vi "Autonomous Independent.vi"() -> ()   [LabVIEW 2014]
doc: "This VI is called when autonomous begins, and will automatically be terminated when autonomous ends. You can carry out timed or sensor driven robot movement independently without needing to return to the caller."
uses:
  Robot Global Data.vi
  <vilib>/Rock Robotics/WPI/RobotDrive/WPI_RobotDriveMecanumDrive_Cartesian.vi
  <vilib>/Rock Robotics/Network Tables/SD Write Numeric Array.vi
panel:
  in  "Instructions":T1(array[cluster])
  out "Current Movement, for debugging":T2 {"Z Joystick Value" scale=-1.0..1.0; "Y Joystick Value" scale=1.0..-1.0; "X Joystick Value" scale=-1.0..1.0}
  in  "Array of robot movements":T3(array[cluster]) {"Z Joystick Value" scale=-1.0..1.0; "Y Joystick Value" scale=1.0..-1.0; "X Joystick Value" scale=-1.0..1.0}
  # "Be sure to right-click and choose Data Operations>>Make Current Value default if you want to save the array values with the VI"
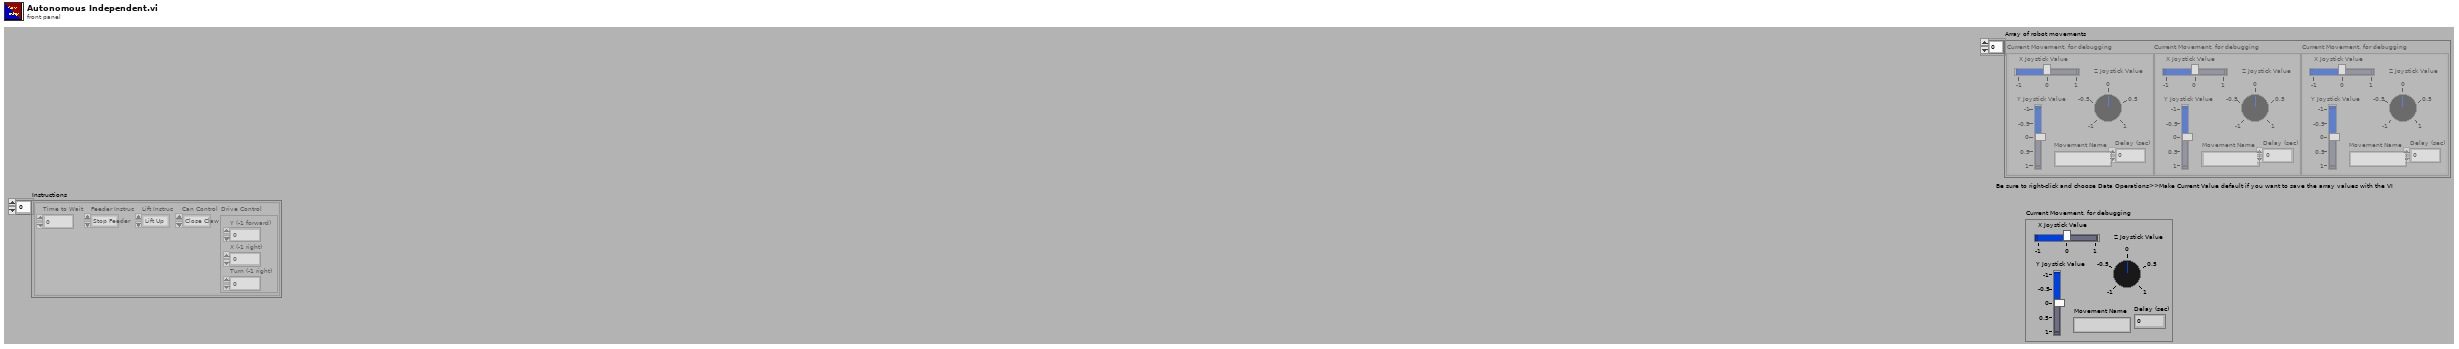
[diagram p1: front panel]
types:
  T1 = cluster{"Time to Wait":dbl, "Feeder Instruc":enum16{"Stop Feeder", "Infeed", "Outfeed", "Rightfeed", "Leftfeed"}, "Lift Instruc":enum16{"Lift Up", "Lift Down"}, "Can Control":enum16{"Close Claw", "Open Claw", "Fast Up", "Slow Up", "Stop", "Srow Down", "Fast Down"}, "Drive Control":cluster{"Y (-1 forward) ":dbl, "X (-1 right)":dbl, "Turn (-1 right)":dbl}}[]
  T2 = cluster{"X Joystick Value":dbl, "Y Joystick Value":dbl, "Z Joystick Value":dbl, "Delay (sec)":dbl, "Movement Name":string}
  T3 = cluster{"X Joystick Value":dbl, "Y Joystick Value":dbl, "Z Joystick Value":dbl, "Delay (sec)":dbl, "Movement Name":string}[]
  T4 = enum16{"open", "replace", "create", "open or create", "replace or create", "replace or create with confirmation"}
  T5 = cluster{"Time to Start":dbl, "Action":enum16{"Stop", "Drive Forward", "Drive Backwards", "Turn Right", "Turn Left", "Tote Up", "Tote Down", "Doors Open", "Doors Close", "Claw Open", "Claw Close", "Claw Up", "Claw Down", "Infeed In", "Infeed Out", "Infeed Off"}}[]
  T6 = typedef "WPI_RobotDriveDevRef.ctl" = cluster{"DevStatus":errorcluster, "Motors[]":T7[], "Square Inputs":bool, "Max Output":dbl}
  T7 = typedef "WPI_MotorControlDeviceRef.ctl" = cluster{"DeviceStatus":errorcluster, "Type":T8, "PWM":cluster{"Controller":T9, "PWM Channel":T10, "DeadBand":T11}, "CAN":cluster{"Device Number":u8, "Control Mode":T12, "Semaphore":T13, "Max Vout":dbl, "TalonSRX Control Mode":T14}, "Invert":bool, "TransformRef":T15, "InvTransformRef":T15}
  T8 = typedef "WPI_MotorControlType.ctl" = enum16{"PWM", "CAN", "CANTalonSRX"}
  T9 = typedef "FPGA_TypedefDigitalModule.ctl" = enum16{"Controller 1"}
  T10 = typedef "FPGA_DIOPWMChannel.ctl" = enum8{"PWM 0", "PWM 1", "PWM 2", "PWM 3", "PWM 4", "PWM 5", "PWM 6", "PWM 7", "PWM 8", "PWM 9", "PWM MXP 0", "PWM MXP 1", "PWM MXP 2", "PWM MXP 3", "PWM MXP 4", "PWM MXP 5", "PWM MXP 6", "PWM MXP 7", "PWM MXP 8", "PWM MXP 9", "Invalid"}
  T11 = typedef "WPI_PWMDeadband.ctl" = cluster{"Name":string, "maxPositivePwm":i32, "minPositivePwm":i32, "centerPwm":i32, "maxNegativePwm":i32, "minNegativePwm":i32, "angularRange":u16}
  T12 = typedef "WPI_CANJaguar_ControlMode.ctl" = enum8{"Percent VBus", "Current", "Speed", "Position", "Voltage"}
  T13 = typedef "Semaphore RefNum" = refnum<k1>
  T14 = typedef "WPI_CANTalonSRX_APIControlMode.ctl" = enum8{"Percent VBus", "Speed", "Position", "Slave", "Unchanged / Invalid"}
  T15 = typedef "WPI_PWMTransform_ConPane.ctl" = refnum<vi>
  T16 = enum16{"Stop Feeder", "Infeed", "Outfeed", "Rightfeed", "Leftfeed"}
  T17 = enum16{"Close Claw", "Open Claw", "Fast Up", "Slow Up", "Stop", "Srow Down", "Fast Down"}
  T18 = cluster{"Y (-1 forward) ":dbl, "X (-1 right)":dbl, "Turn (-1 right)":dbl}
  T19 = cluster{"Lifter Down":bool, "Right Infeed":enum16{"Off", "Forward", "Reverse"}, "Left Infeed":enum16{"Off", "Forward", "Reverse"}}
  T20 = cluster{"Motor Speed":dbl, "Grabber":bool, "Go Up a Level":bool, "Go Down a Level":bool}
  T21 = typedef "Rendezvous RefNum" = refnum<k1>
  T22 = enum16{"Stop", "Drive Forward", "Drive Backwards", "Turn Right", "Turn Left", "Tote Up", "Tote Down", "Doors Open", "Doors Close", "Claw Open", "Claw Close", "Claw Up", "Claw Down", "Infeed In", "Infeed Out", "Infeed Off"}
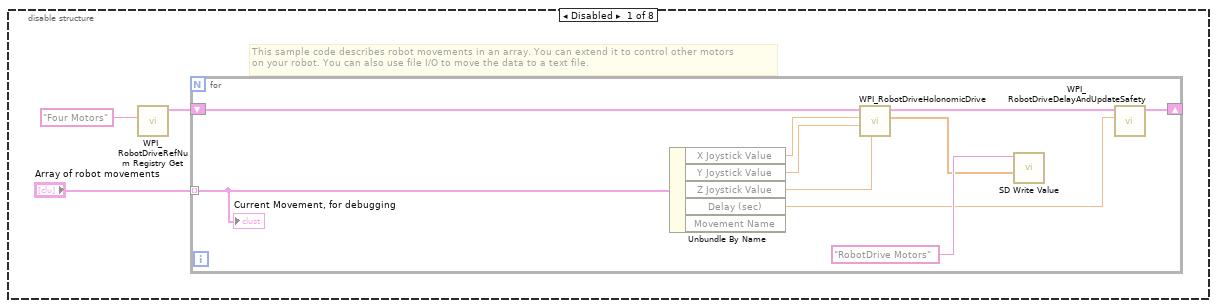
[diagram p2: hidden frame]
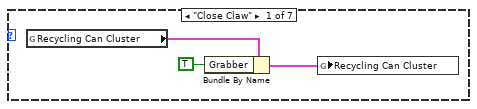
[diagram p3: hidden frame]
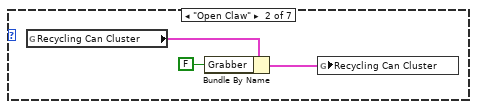
[diagram p4: hidden frame]
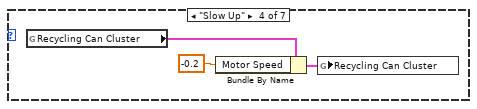
[diagram p5: hidden frame]
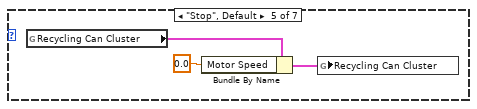
[diagram p6: hidden frame]
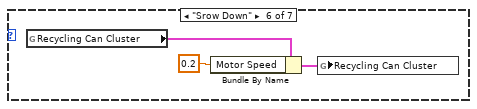
[diagram p7: hidden frame]
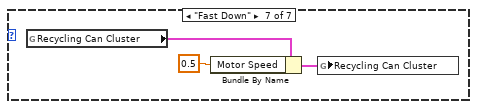
[diagram p8: hidden frame]
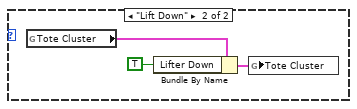
[diagram p9: hidden frame]
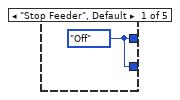
[diagram p10: hidden frame]
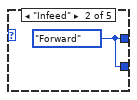
[diagram p11: hidden frame]
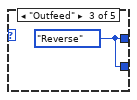
[diagram p12: hidden frame]
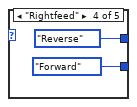
[diagram p13: hidden frame]
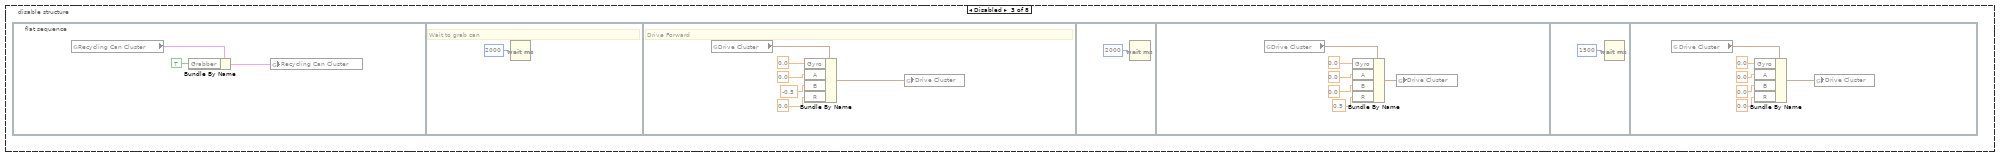
[diagram p14: hidden frame]
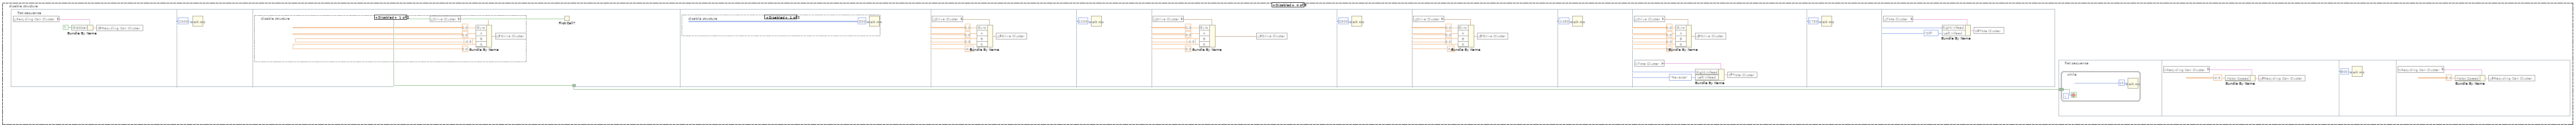
[diagram p15: hidden frame]
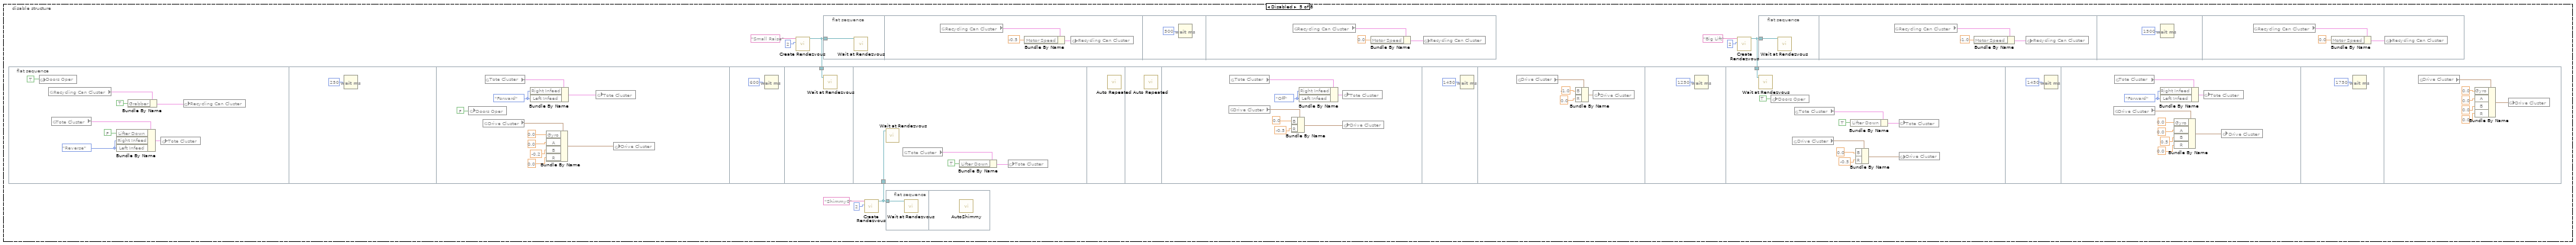
[diagram p18: hidden frame]
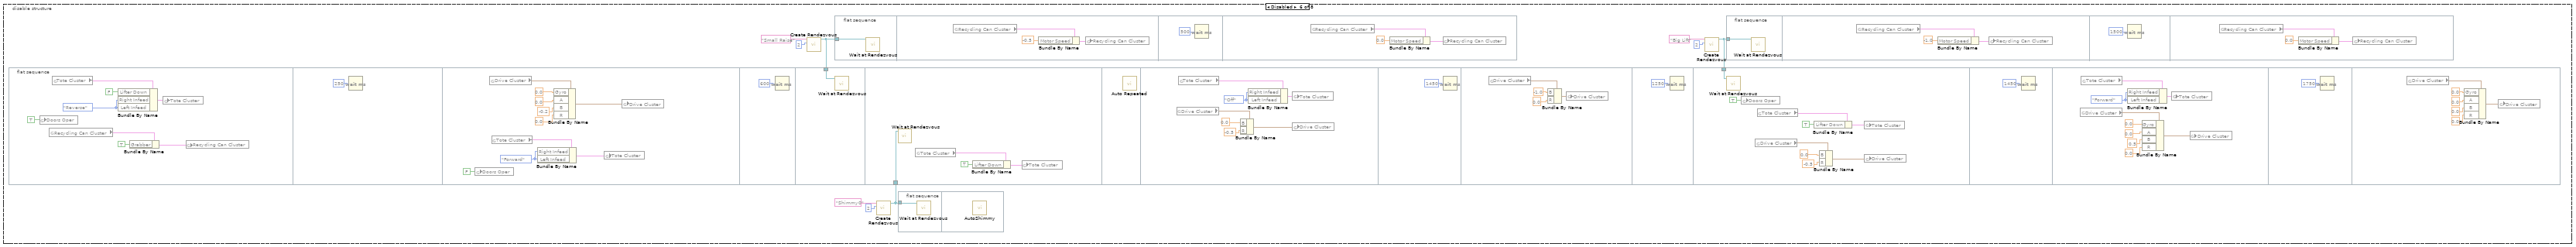
[diagram p19: hidden frame]
diagram:
  # "Every 20ms, report that we are running autonomous\ncode. Loop will abort the same time as the VI."
  # "This tells you the driver position\nand alliance color"
  n1 = call <vilib>:"WPI_DriverStationGet Alliance Info.vi"() -> ()  [unwired: 12 out]
  n2 = disable-structure shown="Enabled" {
    frame Disabled {
      # "This sample code describes robot movements in an array. You can extend it to control other motors\non your robot. You can also use file I/O to move the data to a text file."
      n3 = call <vilib>:"WPI_RobotDriveRefNum Registry Get.vi"("refnum name"="Four Motors") -> ("RobotDriveDevRef"=w2:T6)  [unwired: 1 in, 9 out]
      n4 = for {
        shift-right: [w10] -> _
        shift-left: w2 -> [w11]
        tunnel: "Array of robot movements" -> [w6] mode=indexing
        n5 = Unbundle By Name(w6) -> ("X Joystick Value"=w9:dbl, "Y Joystick Value"=w8:dbl, "Z Joystick Value"=w5:dbl, "Delay (sec)"=w7:dbl)  [unwired: 1 out]
        n6 = call-poly <vilib>:"WPI_RobotDriveHolonomicDrive.vi"("Rotation"=w5, "Y"=w8, "X"=w9, "RobotDriveDevRef"=w11) -> ("Motor Values"=w4:dbl[], "RobotDriveDevRef"=w12:T6)  [unwired: 5 in, 1 out]
        n7 = call-poly <vilib>:"SD Write Value.vi"("Numeric Array"=w4, "Name"="RobotDrive Motors") -> ()  [unwired: 8 in, 2 out]
        n8 = call <vilib>:"WPI_RobotDriveDelayAndUpdateSafety.vi"("Delay (s)"=w7, "RobotDriveDevRef"=w12) -> ("RobotDriveDevRef 2"=w10:T6)  [unwired: 8 in, 1 out]
        "Current Movement, for debugging" <- w6
      }
    }
    frame Enabled {
      n9 = Current VI's Path() -> (path=w21:path)
      n10 = Strip Path(path=w21) -> (stripped path=w22:path)  [unwired: 1 out]
      n11 = Build Path(base path=w22, name or relative path="auto.instruct") -> (appended path=w19:path)
      n12 = Open/Create/Replace File(file path (use dialog)=w19, operation (0:open)=T4."open", access (0:read/write)=enum16{"read/write", "read-only", "write-only"}."read-only") -> (refnum out=w18:refnum<file>)  [unwired: 3 in, 2 out]
      n13 = Read from Text File(file (use dialog)=w18) -> (text=w17:string)  [unwired: 3 in, 3 out]
      n14 = Unflatten From String(type="Instructions", binary string=w17) -> (value=w16:T1)  [unwired: 3 in, 2 out]
      n15 = Array Size(array=w16) -> (size(s)=w20:i32)
      n16 = Tick Count (ms)() -> (millisecond timer value=w14:u32)
      n17 = for {
        N: w20 -> [_]
        tunnel: w16 -> [w32] mode=indexing
        tunnel: w14 -> [w26]
        n18 = Unbundle By Name(w32) -> ("Time to Wait"=w31:dbl, "Feeder Instruc"=w29:T16, "Lift Instruc"=w28:enum16{"Lift Up", "Lift Down"}, "Can Control"=w27:T17, "Drive Control"=w30:T18)
        n19 = flat-sequence {
          tunnel: w31 -> [w33]
          tunnel: w26 -> [w34]
          tunnel: w30 -> [w44]
          tunnel: w29 -> [w43]
          tunnel: w28 -> [w42]
          tunnel: w27 -> [w41]
          frame #0 {
            n20 = while {
              tunnel: w34 -> [w39]
              tunnel: w33 -> [w37]
              stop <- w36 stop-if-true
              n21 = Tick Count (ms)() -> (millisecond timer value=w40:u32)
              n22 = Subtract(x=w40, y=w39) -> (x-y=w38:u32)
              n23 = Greater?(x=w38, y=w37) -> (0:w36:bool)
              n24 = Wait (ms)(milliseconds to wait=u32 5) -> ()  [unwired: 1 out]
            }
          }
          frame #1 {
            n25 = flat-sequence "Feeder Control" {
              tunnel: w43 -> [w78]
              frame #0 {
                n26 = case shown="\"Leftfeed\"" w78 {
                  tunnel: [w79 w80 w81 enum16{"Off", "Forward", "Reverse"}."Reverse" ("Right Infeed") enum16{"Off", "Forward", "Reverse"}."Forward" ("Right Infeed")] -> w75
                  tunnel: [w79 w80 w81 enum16{"Off", "Forward", "Reverse"}."Forward" ("Right Infeed") enum16{"Off", "Forward", "Reverse"}."Reverse" ("Right Infeed")] -> w74
                  frame "Stop Feeder", Default {
                    w79 = enum16{"Off", "Forward", "Reverse"}."Off" ("Right Infeed")
                  }
                  frame "Infeed" {
                    w80 = enum16{"Off", "Forward", "Reverse"}."Forward" ("Right Infeed")
                  }
                  frame "Outfeed" {
                    w81 = enum16{"Off", "Forward", "Reverse"}."Reverse" ("Right Infeed")
                  }
                  frame "Rightfeed" {
                  }
                  frame "Leftfeed" {
                  }
                }
                n27 = global read "Robot Global Data.vi" "Tote Cluster"() -> (w77:T19)
                n28 = Bundle By Name(cluster=w77, "Right Infeed"=w75, "Left Infeed"=w74) -> (w76:T19)
                n29 = global write "Robot Global Data.vi" "Tote Cluster"(w76) -> ()
              }
            }
            n30 = flat-sequence "Lift Instruc" {
              tunnel: w42 -> [w67]
              frame #0 {
                n31 = case shown="\"Lift Up\", Default" w67 {
                  frame "Lift Up", Default {
                    n32 = global read "Robot Global Data.vi" "Tote Cluster"() -> (w70:T19)
                    n33 = Bundle By Name(cluster=w70, "Lifter Down"=FALSE) -> (w69:T19)
                    n34 = global write "Robot Global Data.vi" "Tote Cluster"(w69) -> ()
                  }
                  frame "Lift Down" {
                    n35 = global read "Robot Global Data.vi" "Tote Cluster"() -> (w73:T19)
                    n36 = Bundle By Name(cluster=w73, "Lifter Down"=TRUE) -> (w72:T19)
                    n37 = global write "Robot Global Data.vi" "Tote Cluster"(w72) -> ()
                  }
                }
              }
            }
            n38 = flat-sequence "Claw Instruc" {
              tunnel: w41 -> [w45]
              frame #0 {
                n39 = case shown="\"Fast Up\"" w45 {
                  frame "Close Claw" {
                    n40 = global read "Robot Global Data.vi" "Recycling Can Cluster"() -> (w48:T20)
                    n41 = Bundle By Name(cluster=w48, "Grabber"=TRUE) -> (w47:T20)
                    n42 = global write "Robot Global Data.vi" "Recycling Can Cluster"(w47) -> ()
                  }
                  frame "Open Claw" {
                    n43 = global read "Robot Global Data.vi" "Recycling Can Cluster"() -> (w51:T20)
                    n44 = Bundle By Name(cluster=w51, "Grabber"=FALSE) -> (w50:T20)
                    n45 = global write "Robot Global Data.vi" "Recycling Can Cluster"(w50) -> ()
                  }
                  frame "Fast Up" {
                    n46 = global read "Robot Global Data.vi" "Recycling Can Cluster"() -> (w54:T20)
                    n47 = Bundle By Name(cluster=w54, "Motor Speed"=-0.5) -> (w53:T20)
                    n48 = global write "Robot Global Data.vi" "Recycling Can Cluster"(w53) -> ()
                  }
                  frame "Slow Up" {
                    n49 = global read "Robot Global Data.vi" "Recycling Can Cluster"() -> (w57:T20)
                    n50 = Bundle By Name(cluster=w57, "Motor Speed"=-0.2) -> (w56:T20)
                    n51 = global write "Robot Global Data.vi" "Recycling Can Cluster"(w56) -> ()
                  }
                  frame "Stop", Default {
                    n52 = global read "Robot Global Data.vi" "Recycling Can Cluster"() -> (w60:T20)
                    n53 = Bundle By Name(cluster=w60, "Motor Speed"=0.0) -> (w59:T20)
                    n54 = global write "Robot Global Data.vi" "Recycling Can Cluster"(w59) -> ()
                  }
                  frame "Srow Down" {
                    n55 = global read "Robot Global Data.vi" "Recycling Can Cluster"() -> (w63:T20)
                    n56 = Bundle By Name(cluster=w63, "Motor Speed"=0.2) -> (w62:T20)
                    n57 = global write "Robot Global Data.vi" "Recycling Can Cluster"(w62) -> ()
                  }
                  frame "Fast Down" {
                    n58 = global read "Robot Global Data.vi" "Recycling Can Cluster"() -> (w66:T20)
                    n59 = Bundle By Name(cluster=w66, "Motor Speed"=0.5) -> (w65:T20)
                    n60 = global write "Robot Global Data.vi" "Recycling Can Cluster"(w65) -> ()
                  }
                }
              }
            }
            n61 = flat-sequence "Drive Instruction" {
              tunnel: w44 -> [w91]
              frame #0 {
                n62 = Unbundle By Name(w91) -> ("Y (-1 forward)"=w90:dbl, "X (-1 right)"=w89:dbl, "Turn (-1 right)"=w88:dbl)
                n63 = global read "Robot Global Data.vi" "Drive Cluster"() -> (w87:cluster{"A":dbl, "B":dbl, "R":dbl, "Gyro":dbl})
                n64 = Bundle By Name(cluster=w87, "A"=w89, "B"=w90, "R"=w88) -> (w86:cluster{"A":dbl, "B":dbl, "R":dbl, "Gyro":dbl})
                n65 = global write "Robot Global Data.vi" "Drive Cluster"(w86) -> ()
              }
            }
          }
        }
      }
    }
    frame Disabled {
      n66 = flat-sequence {
        frame #0 {
          n67 = global read "Robot Global Data.vi" "Recycling Can Cluster"() -> (w93:T20)
          n68 = Bundle By Name(cluster=w93, "Grabber"=TRUE) -> (w92:T20)
          n69 = global write "Robot Global Data.vi" "Recycling Can Cluster"(w92) -> ()
        }
        frame #1 {
          # "Wait to grab can"
          n70 = Wait (ms)(milliseconds to wait=u32 2000) -> ()  [unwired: 1 out]
        }
        frame #2 {
          # "Drive Forward"
          n71 = global read "Robot Global Data.vi" "Drive Cluster"() -> (w101:cluster{"A":dbl, "B":dbl, "R":dbl, "Gyro":dbl})
          n72 = Bundle By Name(cluster=w101, "Gyro"=0.0, "A"=0.0, "B"=-0.5, "R"=0.0) -> (w100:cluster{"A":dbl, "B":dbl, "R":dbl, "Gyro":dbl})
          n73 = global write "Robot Global Data.vi" "Drive Cluster"(w100) -> ()
        }
        frame #3 {
          n74 = Wait (ms)(milliseconds to wait=u32 2000 ("millisecond multiple")) -> ()  [unwired: 1 out]
        }
        frame #4 {
          n75 = global read "Robot Global Data.vi" "Drive Cluster"() -> (w103:cluster{"A":dbl, "B":dbl, "R":dbl, "Gyro":dbl})
          n76 = Bundle By Name(cluster=w103, "Gyro"=0.0, "A"=0.0, "B"=0.0, "R"=0.5) -> (w104:cluster{"A":dbl, "B":dbl, "R":dbl, "Gyro":dbl})
          n77 = global write "Robot Global Data.vi" "Drive Cluster"(w104) -> ()
        }
        frame #5 {
          n78 = Wait (ms)(milliseconds to wait=u32 1500 ("millisecond multiple")) -> ()  [unwired: 1 out]
        }
        frame #6 {
          n79 = global read "Robot Global Data.vi" "Drive Cluster"() -> (w110:cluster{"A":dbl, "B":dbl, "R":dbl, "Gyro":dbl})
          n80 = Bundle By Name(cluster=w110, "Gyro"=0.0, "A"=0.0, "B"=0.0, "R"=0.0) -> (w111:cluster{"A":dbl, "B":dbl, "R":dbl, "Gyro":dbl})
          n81 = global write "Robot Global Data.vi" "Drive Cluster"(w111) -> ()
        }
      }
    }
    frame Disabled {
      n82 = flat-sequence {
        tunnel: [w131] -> w116
        frame #0 {
          n83 = global read "Robot Global Data.vi" "Recycling Can Cluster"() -> (w128:T20)
          n84 = Bundle By Name(cluster=w128, "Grabber"=TRUE) -> (w127:T20)
          n85 = global write "Robot Global Data.vi" "Recycling Can Cluster"(w127) -> ()
        }
        frame #1 {
          n86 = Wait (ms)(milliseconds to wait=u32 2000) -> ()  [unwired: 1 out]
        }
        frame #2 {
          n87 = disable-structure shown="Disabled" {
            frame Disabled {
              n88 = global read "Robot Global Data.vi" "Drive Cluster"() -> (w137:cluster{"A":dbl, "B":dbl, "R":dbl, "Gyro":dbl})
              n89 = Bundle By Name(cluster=w137, "Gyro"=0.0, "A"=0.0, "B"=-0.5, "R"=0.0) -> (w136:cluster{"A":dbl, "B":dbl, "R":dbl, "Gyro":dbl})
              n90 = global write "Robot Global Data.vi" "Drive Cluster"(w136) -> ()
            }
            frame Enabled {
            }
          }
          n91 = First Call?() -> (First Call?: T/F=w131:bool)
        }
        frame #3 {
          n92 = disable-structure shown="Disabled" {
            frame Disabled {
              n93 = Wait (ms)(milliseconds to wait=u32 300) -> ()  [unwired: 1 out]
            }
            frame Enabled {
            }
          }
        }
        frame #4 {
          n94 = global read "Robot Global Data.vi" "Drive Cluster"() -> (w140:cluster{"A":dbl, "B":dbl, "R":dbl, "Gyro":dbl})
          n95 = Bundle By Name(cluster=w140, "Gyro"=0.0, "A"=0.0, "B"=0.0, "R"=-0.5) -> (w141:cluster{"A":dbl, "B":dbl, "R":dbl, "Gyro":dbl})
          n96 = global write "Robot Global Data.vi" "Drive Cluster"(w141) -> ()
        }
        frame #5 {
          n97 = Wait (ms)(milliseconds to wait=u32 1200 ("millisecond multiple")) -> ()  [unwired: 1 out]
        }
        frame #6 {
          n98 = global read "Robot Global Data.vi" "Drive Cluster"() -> (w146:cluster{"A":dbl, "B":dbl, "R":dbl, "Gyro":dbl})
          n99 = Bundle By Name(cluster=w146, "Gyro"=0.0, "A"=0.0, "B"=-0.5, "R"=0.0) -> (w147:cluster{"A":dbl, "B":dbl, "R":dbl, "Gyro":dbl})
          n100 = global write "Robot Global Data.vi" "Drive Cluster"(w147) -> ()
        }
        frame #7 {
          n101 = Wait (ms)(milliseconds to wait=u32 2500 ("millisecond multiple")) -> ()  [unwired: 1 out]
        }
        frame #8 {
          n102 = global read "Robot Global Data.vi" "Drive Cluster"() -> (w153:cluster{"A":dbl, "B":dbl, "R":dbl, "Gyro":dbl})
          n103 = Bundle By Name(cluster=w153, "Gyro"=0.0, "A"=0.0, "B"=0.0, "R"=0.5) -> (w154:cluster{"A":dbl, "B":dbl, "R":dbl, "Gyro":dbl})
          n104 = global write "Robot Global Data.vi" "Drive Cluster"(w154) -> ()
        }
        frame #9 {
          n105 = Wait (ms)(milliseconds to wait=u32 1450 ("millisecond multiple")) -> ()  [unwired: 1 out]
        }
        frame #10 {
          w160 = enum16{"Off", "Forward", "Reverse"}."Reverse" ("Right Infeed")
          n106 = global read "Robot Global Data.vi" "Drive Cluster"() -> (w168:cluster{"A":dbl, "B":dbl, "R":dbl, "Gyro":dbl})
          n107 = global read "Robot Global Data.vi" "Tote Cluster"() -> (w161:T19)
          n108 = Bundle By Name(cluster=w168, "Gyro"=0.0, "A"=0.0, "B"=0.0, "R"=0.0) -> (w167:cluster{"A":dbl, "B":dbl, "R":dbl, "Gyro":dbl})
          n109 = global write "Robot Global Data.vi" "Drive Cluster"(w167) -> ()
          n110 = Bundle By Name(cluster=w161, "Right Infeed"=w160, "Left Infeed"=w160) -> (w162:T19)
          n111 = global write "Robot Global Data.vi" "Tote Cluster"(w162) -> ()
        }
        frame #11 {
          n112 = Wait (ms)(milliseconds to wait=u32 1750 ("millisecond multiple")) -> ()  [unwired: 1 out]
        }
        frame #12 {
          w170 = enum16{"Off", "Forward", "Reverse"}."Off" ("Right Infeed")
          n113 = global read "Robot Global Data.vi" "Tote Cluster"() -> (w171:T19)
          n114 = Bundle By Name(cluster=w171, "Right Infeed"=w170, "Left Infeed"=w170) -> (w172:T19)
          n115 = global write "Robot Global Data.vi" "Tote Cluster"(w172) -> ()
        }
      }
      n116 = flat-sequence {
        tunnel: w116 -> [w117]
        frame #0 {
          n117 = while {
            tunnel: w117 -> [w119]
            stop <- w119 stop-if-true
            n118 = Wait (ms)(milliseconds to wait=u32 10) -> ()  [unwired: 1 out]
          }
        }
        frame #1 {
          n119 = global read "Robot Global Data.vi" "Recycling Can Cluster"() -> (w121:T20)
          n120 = Bundle By Name(cluster=w121, "Motor Speed"=-0.5) -> (w120:T20)
          n121 = global write "Robot Global Data.vi" "Recycling Can Cluster"(w120) -> ()
        }
        frame #2 {
          n122 = Wait (ms)(milliseconds to wait=u32 500) -> ()  [unwired: 1 out]
        }
        frame #3 {
          n123 = global read "Robot Global Data.vi" "Recycling Can Cluster"() -> (w125:T20)
          n124 = Bundle By Name(cluster=w125, "Motor Speed"=0.0) -> (w124:T20)
          n125 = global write "Robot Global Data.vi" "Recycling Can Cluster"(w124) -> ()
        }
      }
    }
    frame Disabled {
      n126 = flat-sequence {
        tunnel: w179 -> [w211]
        tunnel: w173 -> [w212]
        tunnel: w177 -> [w232]
        frame #0 {
          w193 = enum16{"Off", "Forward", "Reverse"}."Reverse" ("Right Infeed")
          n127 = global write "Robot Global Data.vi" "Doors Oper"(TRUE ("Doors Oper")) -> ()
          n128 = global read "Robot Global Data.vi" "Recycling Can Cluster"() -> (w197:T20)
          n129 = global read "Robot Global Data.vi" "Tote Cluster"() -> (w192:T19)
          n130 = Bundle By Name(cluster=w192, "Lifter Down"=FALSE ("Lifter"), "Right Infeed"=w193, "Left Infeed"=w193) -> (w191:T19)
          n131 = Bundle By Name(cluster=w197, "Grabber"=TRUE) -> (w196:T20)
          n132 = global write "Robot Global Data.vi" "Tote Cluster"(w191) -> ()
          n133 = global write "Robot Global Data.vi" "Recycling Can Cluster"(w196) -> ()
        }
        frame #1 {
          n134 = Wait (ms)(milliseconds to wait=u32 250) -> ()  [unwired: 1 out]
        }
        frame #2 {
          w207 = enum16{"Off", "Forward", "Reverse"}."Forward" ("Right Infeed")
          n135 = global write "Robot Global Data.vi" "Doors Oper"(FALSE ("Doors Oper")) -> ()
          n136 = global read "Robot Global Data.vi" "Drive Cluster"() -> (w204:cluster{"A":dbl, "B":dbl, "R":dbl, "Gyro":dbl})
          n137 = global read "Robot Global Data.vi" "Tote Cluster"() -> (w208:T19)
          n138 = Bundle By Name(cluster=w208, "Right Infeed"=w207, "Left Infeed"=w207) -> (w209:T19)
          n139 = Bundle By Name(cluster=w204, "Gyro"=0.0, "A"=0.0, "B"=-0.2, "R"=0.0) -> (w203:cluster{"A":dbl, "B":dbl, "R":dbl, "Gyro":dbl})
          n140 = global write "Robot Global Data.vi" "Tote Cluster"(w209) -> ()
          n141 = global write "Robot Global Data.vi" "Drive Cluster"(w203) -> ()
        }
        frame #3 {
          n142 = Wait (ms)(milliseconds to wait=u32 600) -> ()  [unwired: 1 out]
        }
        frame #4 {
          n143 = call <vilib>:"Wait at Rendezvous.vi"("rendezvous"=w211) -> ()  [unwired: 4 in, 3 out]
        }
        frame #5 {
          n144 = call <vilib>:"Wait at Rendezvous.vi"("rendezvous"=w212) -> ()  [unwired: 4 in, 3 out]
          n145 = global read "Robot Global Data.vi" "Tote Cluster"() -> (w213:T19)
          n146 = Bundle By Name(cluster=w213, "Lifter Down"=TRUE ("Lifter")) -> (w214:T19)
          n147 = global write "Robot Global Data.vi" "Tote Cluster"(w214) -> ()
        }
        frame #6 {
          n148 = call "Auto Repeated.vi"() -> ()  [unwired: 12 in]
        }
        frame #7 {
          n149 = call "Auto Repeated.vi"() -> ()  [unwired: 12 in]
        }
        frame #8 {
          w218 = enum16{"Off", "Forward", "Reverse"}."Off" ("Right Infeed")
          n150 = global read "Robot Global Data.vi" "Drive Cluster"() -> (w222:cluster{"A":dbl, "B":dbl, "R":dbl, "Gyro":dbl})
          n151 = global read "Robot Global Data.vi" "Tote Cluster"() -> (w217:T19)
          n152 = Bundle By Name(cluster=w222, "B"=0.0, "R"=-0.5) -> (w221:cluster{"A":dbl, "B":dbl, "R":dbl, "Gyro":dbl})
          n153 = Bundle By Name(cluster=w217, "Right Infeed"=w218, "Left Infeed"=w218) -> (w216:T19)
          n154 = global write "Robot Global Data.vi" "Tote Cluster"(w216) -> ()
          n155 = global write "Robot Global Data.vi" "Drive Cluster"(w221) -> ()
        }
        frame #9 {
          n156 = Wait (ms)(milliseconds to wait=u32 1450 ("millisecond multiple")) -> ()  [unwired: 1 out]
        }
        frame #10 {
          n157 = global read "Robot Global Data.vi" "Drive Cluster"() -> (w225:cluster{"A":dbl, "B":dbl, "R":dbl, "Gyro":dbl})
          n158 = Bundle By Name(cluster=w225, "B"=-1.0, "R"=0.0) -> (w226:cluster{"A":dbl, "B":dbl, "R":dbl, "Gyro":dbl})
          n159 = global write "Robot Global Data.vi" "Drive Cluster"(w226) -> ()
        }
        frame #11 {
          n160 = Wait (ms)(milliseconds to wait=u32 1250 ("millisecond multiple")) -> ()  [unwired: 1 out]
        }
        frame #12 {
          n161 = call <vilib>:"Wait at Rendezvous.vi"("rendezvous"=w232) -> ()  [unwired: 4 in, 3 out]
          n162 = global write "Robot Global Data.vi" "Doors Oper"(TRUE ("Doors Oper")) -> ()
          n163 = global read "Robot Global Data.vi" "Drive Cluster"() -> (w234:cluster{"A":dbl, "B":dbl, "R":dbl, "Gyro":dbl})
          n164 = global read "Robot Global Data.vi" "Tote Cluster"() -> (w230:T19)
          n165 = Bundle By Name(cluster=w230, "Lifter Down"=TRUE ("Lifter")) -> (w231:T19)
          n166 = Bundle By Name(cluster=w234, "B"=0.0, "R"=-0.5) -> (w235:cluster{"A":dbl, "B":dbl, "R":dbl, "Gyro":dbl})
          n167 = global write "Robot Global Data.vi" "Tote Cluster"(w231) -> ()
          n168 = global write "Robot Global Data.vi" "Drive Cluster"(w235) -> ()
        }
        frame #13 {
          n169 = Wait (ms)(milliseconds to wait=u32 1450 ("millisecond multiple")) -> ()  [unwired: 1 out]
        }
        frame #14 {
          w239 = enum16{"Off", "Forward", "Reverse"}."Forward" ("Right Infeed")
          n170 = global read "Robot Global Data.vi" "Drive Cluster"() -> (w247:cluster{"A":dbl, "B":dbl, "R":dbl, "Gyro":dbl})
          n171 = global read "Robot Global Data.vi" "Tote Cluster"() -> (w240:T19)
          n172 = Bundle By Name(cluster=w240, "Right Infeed"=w239, "Left Infeed"=w239) -> (w241:T19)
          n173 = Bundle By Name(cluster=w247, "Gyro"=0.0, "A"=0.0, "B"=0.5, "R"=0.0) -> (w246:cluster{"A":dbl, "B":dbl, "R":dbl, "Gyro":dbl})
          n174 = global write "Robot Global Data.vi" "Tote Cluster"(w241) -> ()
          n175 = global write "Robot Global Data.vi" "Drive Cluster"(w246) -> ()
        }
        frame #15 {
          n176 = Wait (ms)(milliseconds to wait=u32 1750 ("millisecond multiple")) -> ()  [unwired: 1 out]
        }
        frame #16 {
          n177 = global read "Robot Global Data.vi" "Drive Cluster"() -> (w249:cluster{"A":dbl, "B":dbl, "R":dbl, "Gyro":dbl})
          n178 = Bundle By Name(cluster=w249, "Gyro"=0.0, "A"=0.0, "B"=0.0, "R"=0.0) -> (w250:cluster{"A":dbl, "B":dbl, "R":dbl, "Gyro":dbl})
          n179 = global write "Robot Global Data.vi" "Drive Cluster"(w250) -> ()
        }
      }
      n180 = call <vilib>:"Create Rendezvous.vi"("size (2)"=2, "name (unnamed)"="Small Raise") -> ("rendezvous"=w179:T21)  [unwired: 3 in, 2 out]
      n181 = flat-sequence {
        tunnel: w179 -> [w255]
        frame #0 {
          n182 = call <vilib>:"Wait at Rendezvous.vi"("rendezvous"=w255) -> ()  [unwired: 4 in, 3 out]
        }
        frame #1 {
          n183 = global read "Robot Global Data.vi" "Recycling Can Cluster"() -> (w257:T20)
          n184 = Bundle By Name(cluster=w257, "Motor Speed"=-0.5) -> (w256:T20)
          n185 = global write "Robot Global Data.vi" "Recycling Can Cluster"(w256) -> ()
        }
        frame #2 {
          n186 = Wait (ms)(milliseconds to wait=u32 500) -> ()  [unwired: 1 out]
        }
        frame #3 {
          n187 = global read "Robot Global Data.vi" "Recycling Can Cluster"() -> (w261:T20)
          n188 = Bundle By Name(cluster=w261, "Motor Speed"=0.0) -> (w260:T20)
          n189 = global write "Robot Global Data.vi" "Recycling Can Cluster"(w260) -> ()
        }
      }
      n190 = call <vilib>:"Create Rendezvous.vi"("size (2)"=2, "name (unnamed)"="Shimmy0") -> ("rendezvous"=w173:T21)  [unwired: 3 in, 2 out]
      n191 = flat-sequence {
        tunnel: w173 -> [w182]
        frame #0 {
          n192 = call <vilib>:"Wait at Rendezvous.vi"("rendezvous"=w182) -> ()  [unwired: 4 in, 3 out]
        }
        frame #1 {
          n193 = call "AutoShimmy.vi"() -> ()  [unwired: 12 in]
        }
      }
      n194 = call <vilib>:"Create Rendezvous.vi"("size (2)"=2, "name (unnamed)"="Big Lift") -> ("rendezvous"=w177:T21)  [unwired: 3 in, 2 out]
      n195 = flat-sequence {
        tunnel: w177 -> [w183]
        frame #0 {
          n196 = call <vilib>:"Wait at Rendezvous.vi"("rendezvous"=w183) -> ()  [unwired: 4 in, 3 out]
        }
        frame #1 {
          n197 = global read "Robot Global Data.vi" "Recycling Can Cluster"() -> (w185:T20)
          n198 = Bundle By Name(cluster=w185, "Motor Speed"=-1.0) -> (w184:T20)
          n199 = global write "Robot Global Data.vi" "Recycling Can Cluster"(w184) -> ()
        }
        frame #2 {
          n200 = Wait (ms)(milliseconds to wait=u32 1500) -> ()  [unwired: 1 out]
        }
        frame #3 {
          n201 = global read "Robot Global Data.vi" "Recycling Can Cluster"() -> (w189:T20)
          n202 = Bundle By Name(cluster=w189, "Motor Speed"=0.0) -> (w188:T20)
          n203 = global write "Robot Global Data.vi" "Recycling Can Cluster"(w188) -> ()
        }
      }
    }
    frame Disabled {
      n204 = flat-sequence {
        tunnel: w269 -> [w301]
        tunnel: w263 -> [w302]
        tunnel: w267 -> [w322]
        frame #0 {
          w283 = enum16{"Off", "Forward", "Reverse"}."Reverse" ("Right Infeed")
          n205 = global write "Robot Global Data.vi" "Doors Oper"(TRUE ("Doors Oper")) -> ()
          n206 = global read "Robot Global Data.vi" "Recycling Can Cluster"() -> (w287:T20)
          n207 = global read "Robot Global Data.vi" "Tote Cluster"() -> (w282:T19)
          n208 = Bundle By Name(cluster=w282, "Lifter Down"=FALSE ("Lifter"), "Right Infeed"=w283, "Left Infeed"=w283) -> (w281:T19)
          n209 = Bundle By Name(cluster=w287, "Grabber"=TRUE) -> (w286:T20)
          n210 = global write "Robot Global Data.vi" "Tote Cluster"(w281) -> ()
          n211 = global write "Robot Global Data.vi" "Recycling Can Cluster"(w286) -> ()
        }
        frame #1 {
          n212 = Wait (ms)(milliseconds to wait=u32 250) -> ()  [unwired: 1 out]
        }
        frame #2 {
          w297 = enum16{"Off", "Forward", "Reverse"}."Forward" ("Right Infeed")
          n213 = global write "Robot Global Data.vi" "Doors Oper"(FALSE ("Doors Oper")) -> ()
          n214 = global read "Robot Global Data.vi" "Drive Cluster"() -> (w294:cluster{"A":dbl, "B":dbl, "R":dbl, "Gyro":dbl})
          n215 = global read "Robot Global Data.vi" "Tote Cluster"() -> (w298:T19)
          n216 = Bundle By Name(cluster=w298, "Right Infeed"=w297, "Left Infeed"=w297) -> (w299:T19)
          n217 = Bundle By Name(cluster=w294, "Gyro"=0.0, "A"=0.0, "B"=-0.2, "R"=0.0) -> (w293:cluster{"A":dbl, "B":dbl, "R":dbl, "Gyro":dbl})
          n218 = global write "Robot Global Data.vi" "Tote Cluster"(w299) -> ()
          n219 = global write "Robot Global Data.vi" "Drive Cluster"(w293) -> ()
        }
        frame #3 {
          n220 = Wait (ms)(milliseconds to wait=u32 600) -> ()  [unwired: 1 out]
        }
        frame #4 {
          n221 = call <vilib>:"Wait at Rendezvous.vi"("rendezvous"=w301) -> ()  [unwired: 4 in, 3 out]
        }
        frame #5 {
          n222 = call <vilib>:"Wait at Rendezvous.vi"("rendezvous"=w302) -> ()  [unwired: 4 in, 3 out]
          n223 = global read "Robot Global Data.vi" "Tote Cluster"() -> (w303:T19)
          n224 = Bundle By Name(cluster=w303, "Lifter Down"=TRUE ("Lifter")) -> (w304:T19)
          n225 = global write "Robot Global Data.vi" "Tote Cluster"(w304) -> ()
        }
        frame #6 {
          n226 = call "Auto Repeated.vi"() -> ()  [unwired: 12 in]
        }
        frame #7 {
          w308 = enum16{"Off", "Forward", "Reverse"}."Off" ("Right Infeed")
          n227 = global read "Robot Global Data.vi" "Drive Cluster"() -> (w312:cluster{"A":dbl, "B":dbl, "R":dbl, "Gyro":dbl})
          n228 = global read "Robot Global Data.vi" "Tote Cluster"() -> (w307:T19)
          n229 = Bundle By Name(cluster=w312, "B"=0.0, "R"=-0.5) -> (w311:cluster{"A":dbl, "B":dbl, "R":dbl, "Gyro":dbl})
          n230 = Bundle By Name(cluster=w307, "Right Infeed"=w308, "Left Infeed"=w308) -> (w306:T19)
          n231 = global write "Robot Global Data.vi" "Tote Cluster"(w306) -> ()
          n232 = global write "Robot Global Data.vi" "Drive Cluster"(w311) -> ()
        }
        frame #8 {
          n233 = Wait (ms)(milliseconds to wait=u32 1450 ("millisecond multiple")) -> ()  [unwired: 1 out]
        }
        frame #9 {
          n234 = global read "Robot Global Data.vi" "Drive Cluster"() -> (w315:cluster{"A":dbl, "B":dbl, "R":dbl, "Gyro":dbl})
          n235 = Bundle By Name(cluster=w315, "B"=-1.0, "R"=0.0) -> (w316:cluster{"A":dbl, "B":dbl, "R":dbl, "Gyro":dbl})
          n236 = global write "Robot Global Data.vi" "Drive Cluster"(w316) -> ()
        }
        frame #10 {
          n237 = Wait (ms)(milliseconds to wait=u32 1250 ("millisecond multiple")) -> ()  [unwired: 1 out]
        }
        frame #11 {
          n238 = call <vilib>:"Wait at Rendezvous.vi"("rendezvous"=w322) -> ()  [unwired: 4 in, 3 out]
          n239 = global write "Robot Global Data.vi" "Doors Oper"(TRUE ("Doors Oper")) -> ()
          n240 = global read "Robot Global Data.vi" "Drive Cluster"() -> (w324:cluster{"A":dbl, "B":dbl, "R":dbl, "Gyro":dbl})
          n241 = global read "Robot Global Data.vi" "Tote Cluster"() -> (w320:T19)
          n242 = Bundle By Name(cluster=w320, "Lifter Down"=TRUE ("Lifter")) -> (w321:T19)
          n243 = Bundle By Name(cluster=w324, "B"=0.0, "R"=-0.5) -> (w325:cluster{"A":dbl, "B":dbl, "R":dbl, "Gyro":dbl})
          n244 = global write "Robot Global Data.vi" "Tote Cluster"(w321) -> ()
          n245 = global write "Robot Global Data.vi" "Drive Cluster"(w325) -> ()
        }
        frame #12 {
          n246 = Wait (ms)(milliseconds to wait=u32 1450 ("millisecond multiple")) -> ()  [unwired: 1 out]
        }
        frame #13 {
          w329 = enum16{"Off", "Forward", "Reverse"}."Forward" ("Right Infeed")
          n247 = global read "Robot Global Data.vi" "Drive Cluster"() -> (w337:cluster{"A":dbl, "B":dbl, "R":dbl, "Gyro":dbl})
          n248 = global read "Robot Global Data.vi" "Tote Cluster"() -> (w330:T19)
          n249 = Bundle By Name(cluster=w330, "Right Infeed"=w329, "Left Infeed"=w329) -> (w331:T19)
          n250 = Bundle By Name(cluster=w337, "Gyro"=0.0, "A"=0.0, "B"=0.5, "R"=0.0) -> (w336:cluster{"A":dbl, "B":dbl, "R":dbl, "Gyro":dbl})
          n251 = global write "Robot Global Data.vi" "Tote Cluster"(w331) -> ()
          n252 = global write "Robot Global Data.vi" "Drive Cluster"(w336) -> ()
        }
        frame #14 {
          n253 = Wait (ms)(milliseconds to wait=u32 1750 ("millisecond multiple")) -> ()  [unwired: 1 out]
        }
        frame #15 {
          n254 = global read "Robot Global Data.vi" "Drive Cluster"() -> (w339:cluster{"A":dbl, "B":dbl, "R":dbl, "Gyro":dbl})
          n255 = Bundle By Name(cluster=w339, "Gyro"=0.0, "A"=0.0, "B"=0.0, "R"=0.0) -> (w340:cluster{"A":dbl, "B":dbl, "R":dbl, "Gyro":dbl})
          n256 = global write "Robot Global Data.vi" "Drive Cluster"(w340) -> ()
        }
      }
      n257 = call <vilib>:"Create Rendezvous.vi"("size (2)"=2, "name (unnamed)"="Small Raise") -> ("rendezvous"=w269:T21)  [unwired: 3 in, 2 out]
      n258 = flat-sequence {
        tunnel: w269 -> [w345]
        frame #0 {
          n259 = call <vilib>:"Wait at Rendezvous.vi"("rendezvous"=w345) -> ()  [unwired: 4 in, 3 out]
        }
        frame #1 {
          n260 = global read "Robot Global Data.vi" "Recycling Can Cluster"() -> (w347:T20)
          n261 = Bundle By Name(cluster=w347, "Motor Speed"=-0.5) -> (w346:T20)
          n262 = global write "Robot Global Data.vi" "Recycling Can Cluster"(w346) -> ()
        }
        frame #2 {
          n263 = Wait (ms)(milliseconds to wait=u32 500) -> ()  [unwired: 1 out]
        }
        frame #3 {
          n264 = global read "Robot Global Data.vi" "Recycling Can Cluster"() -> (w351:T20)
          n265 = Bundle By Name(cluster=w351, "Motor Speed"=0.0) -> (w350:T20)
          n266 = global write "Robot Global Data.vi" "Recycling Can Cluster"(w350) -> ()
        }
      }
      n267 = call <vilib>:"Create Rendezvous.vi"("size (2)"=2, "name (unnamed)"="Shimmy0") -> ("rendezvous"=w263:T21)  [unwired: 3 in, 2 out]
      n268 = flat-sequence {
        tunnel: w263 -> [w272]
        frame #0 {
          n269 = call <vilib>:"Wait at Rendezvous.vi"("rendezvous"=w272) -> ()  [unwired: 4 in, 3 out]
        }
        frame #1 {
          n270 = call "AutoShimmy.vi"() -> ()  [unwired: 12 in]
        }
      }
      n271 = call <vilib>:"Create Rendezvous.vi"("size (2)"=2, "name (unnamed)"="Big Lift") -> ("rendezvous"=w267:T21)  [unwired: 3 in, 2 out]
      n272 = flat-sequence {
        tunnel: w267 -> [w273]
        frame #0 {
          n273 = call <vilib>:"Wait at Rendezvous.vi"("rendezvous"=w273) -> ()  [unwired: 4 in, 3 out]
        }
        frame #1 {
          n274 = global read "Robot Global Data.vi" "Recycling Can Cluster"() -> (w275:T20)
          n275 = Bundle By Name(cluster=w275, "Motor Speed"=-1.0) -> (w274:T20)
          n276 = global write "Robot Global Data.vi" "Recycling Can Cluster"(w274) -> ()
        }
        frame #2 {
          n277 = Wait (ms)(milliseconds to wait=u32 1500) -> ()  [unwired: 1 out]
        }
        frame #3 {
          n278 = global read "Robot Global Data.vi" "Recycling Can Cluster"() -> (w279:T20)
          n279 = Bundle By Name(cluster=w279, "Motor Speed"=0.0) -> (w278:T20)
          n280 = global write "Robot Global Data.vi" "Recycling Can Cluster"(w278) -> ()
        }
      }
    }
    frame Disabled {
    }
    frame Disabled {
      n281 = Current VI's Path() -> (path=w355:path)
      n282 = Build Path(base path=w355, name or relative path="AutoList.instruct") -> (appended path=w357:path)
      n283 = Read from Binary File(11:w357) -> (0:w353:errorcluster, 2:w354:string)  [unwired: 5 in, 2 out]
      n284 = case shown="No Error" w353 {
        tunnel: w354 -> [w360 _]
        frame No Error {
          n285 = Unflatten From String(type=T5 [] ("Actions"), binary string=w360) -> (value=w358:T5)  [unwired: 3 in, 2 out]
          n286 = Array Size(array=w358) -> (size(s)=w359:i32)
          n287 = for {
            N: w359 -> [_]
            tunnel: w358 -> [w365] mode=indexing
            n288 = Unbundle By Name(w365) -> ("Time to Start"=w364:dbl, "Action"=w362:T22)
            n289 = flat-sequence {
              tunnel: w364 -> [w367]
              tunnel: [w366] -> w363
              tunnel: w362 -> [w366]
              tunnel: w363 -> [w368]
              frame #0 {
                n290 = Wait Until Next ms Multiple(millisecond multiple=w367) -> ()  [unwired: 1 out]
              }
              frame #1 {
                n291 = case shown="\"Doors Close\"" w368 {
                  frame "Stop", Default {
                    n292 = Wait (ms)(milliseconds to wait=u32 50) -> ()  [unwired: 1 out]
                  }
                  frame "Drive Forward" {
                    n293 = global read "Robot Global Data.vi" "Drive Cluster"() -> (w375:cluster{"A":dbl, "B":dbl, "R":dbl, "Gyro":dbl})
                    n294 = Bundle By Name(cluster=w375, "Gyro"=0.0, "A"=0.0, "B"=0.5, "R"=0.0) -> (w374:cluster{"A":dbl, "B":dbl, "R":dbl, "Gyro":dbl})
                    n295 = global write "Robot Global Data.vi" "Drive Cluster"(w374) -> ()
                  }
                  frame "Drive Backwards" {
                    n296 = global read "Robot Global Data.vi" "Drive Cluster"() -> (w376:cluster{"A":dbl, "B":dbl, "R":dbl, "Gyro":dbl})
                    n297 = Bundle By Name(cluster=w376, "Gyro"=0.0, "A"=0.0, "B"=-0.5, "R"=0.0) -> (w377:cluster{"A":dbl, "B":dbl, "R":dbl, "Gyro":dbl})
                    n298 = global write "Robot Global Data.vi" "Drive Cluster"(w377) -> ()
                  }
                  frame "Turn Right" {
                    n299 = global read "Robot Global Data.vi" "Drive Cluster"() -> (w382:cluster{"A":dbl, "B":dbl, "R":dbl, "Gyro":dbl})
                    n300 = Bundle By Name(cluster=w382, "Gyro"=0.0, "A"=0.0, "B"=0.0, "R"=0.5) -> (w383:cluster{"A":dbl, "B":dbl, "R":dbl, "Gyro":dbl})
                    n301 = global write "Robot Global Data.vi" "Drive Cluster"(w383) -> ()
                  }
                  frame "Turn Left" {
                    n302 = global read "Robot Global Data.vi" "Drive Cluster"() -> (w388:cluster{"A":dbl, "B":dbl, "R":dbl, "Gyro":dbl})
                    n303 = Bundle By Name(cluster=w388, "Gyro"=0.0, "A"=0.0, "B"=0.0, "R"=-0.5) -> (w389:cluster{"A":dbl, "B":dbl, "R":dbl, "Gyro":dbl})
                    n304 = global write "Robot Global Data.vi" "Drive Cluster"(w389) -> ()
                  }
                  frame "Tote Up" {
                    n305 = global read "Robot Global Data.vi" "Tote Cluster"() -> (w395:T19)
                    n306 = Bundle By Name(cluster=w395, "Lifter Down"=TRUE ("Lifter")) -> (w396:T19)
                    n307 = global write "Robot Global Data.vi" "Tote Cluster"(w396) -> ()
                  }
                  frame "Tote Down" {
                    n308 = global read "Robot Global Data.vi" "Tote Cluster"() -> (w398:T19)
                    n309 = Bundle By Name(cluster=w398, "Lifter Down"=FALSE ("Lifter")) -> (w399:T19)
                    n310 = global write "Robot Global Data.vi" "Tote Cluster"(w399) -> ()
                  }
                  frame "Doors Open" {
                    n311 = global write "Robot Global Data.vi" "Doors Oper"(TRUE ("Lifter")) -> ()
                  }
                  frame "Doors Close" {
                    n312 = global write "Robot Global Data.vi" "Doors Oper"(FALSE ("Lifter")) -> ()
                  }
                  frame "Claw Open" {
                    n313 = global read "Robot Global Data.vi" "Recycling Can Cluster"() -> (w403:T20)
                    n314 = Bundle By Name(cluster=w403, "Grabber"=TRUE) -> (w402:T20)
                    n315 = global write "Robot Global Data.vi" "Recycling Can Cluster"(w402) -> ()
                  }
                  frame "Claw Close" {
                    n316 = global read "Robot Global Data.vi" "Recycling Can Cluster"() -> (w406:T20)
                    n317 = Bundle By Name(cluster=w406, "Grabber"=FALSE) -> (w407:T20)
                    n318 = global write "Robot Global Data.vi" "Recycling Can Cluster"(w407) -> ()
                  }
                  frame "Claw Up" {
                    n319 = global read "Robot Global Data.vi" "Recycling Can Cluster"() -> (w409:T20)
                    n320 = Bundle By Name(cluster=w409, "Go Up a Level"=TRUE ("Grabber")) -> (w410:T20)
                    n321 = global write "Robot Global Data.vi" "Recycling Can Cluster"(w410) -> ()
                  }
                  frame "Claw Down" {
                    n322 = global read "Robot Global Data.vi" "Recycling Can Cluster"() -> (w412:T20)
                    n323 = Bundle By Name(cluster=w412, "Go Down a Level"=TRUE ("Grabber")) -> (w413:T20)
                    n324 = global write "Robot Global Data.vi" "Recycling Can Cluster"(w413) -> ()
                  }
                  frame "Infeed In" {
                    w414 = enum16{"Off", "Forward", "Reverse"}."Forward" ("Right Infeed")
                    n325 = global read "Robot Global Data.vi" "Tote Cluster"() -> (w415:T19)
                    n326 = Bundle By Name(cluster=w415, "Right Infeed"=w414, "Left Infeed"=w414) -> (w416:T19)
                    n327 = global write "Robot Global Data.vi" "Tote Cluster"(w416) -> ()
                  }
                  frame "Infeed Out" {
                    w417 = enum16{"Off", "Forward", "Reverse"}."Reverse" ("Right Infeed")
                    n328 = global read "Robot Global Data.vi" "Tote Cluster"() -> (w418:T19)
                    n329 = Bundle By Name(cluster=w418, "Right Infeed"=w417, "Left Infeed"=w417) -> (w419:T19)
                    n330 = global write "Robot Global Data.vi" "Tote Cluster"(w419) -> ()
                  }
                  frame "Infeed Off" {
                    w422 = enum16{"Off", "Forward", "Reverse"}."Off" ("Right Infeed")
                    n331 = global read "Robot Global Data.vi" "Tote Cluster"() -> (w421:T19)
                    n332 = Bundle By Name(cluster=w421, "Right Infeed"=w422, "Left Infeed"=w422) -> (w420:T19)
                    n333 = global write "Robot Global Data.vi" "Tote Cluster"(w420) -> ()
                  }
                }
              }
            }
          }
        }
        frame Error {
        }
      }
    }
  }
  n334 = while {
    stop <- FALSE stop-if-true
    n335 = call <vilib>:"WPI_DriverStationReport Robot Code State.vi"("Autonomous"=TRUE) -> ()  [unwired: 10 in, 1 out]
    n336 = Wait (ms)(milliseconds to wait=u32 20) -> ()  [unwired: 1 out]
  }
